vi "FTW-SEQ-Destroy.vi"(1 "FTW Job Sequencer":refnum<class "FTW-JobSequencer.lvclass">) -> ()   [LabVIEW 2012, in "FTW-Actor.lvlib" / "FTW-JobSequencer.lvclass"]
uses:
  FTW-JobSequencer.lvclass
panel:
  # "Inputs"
  # "Outputs"
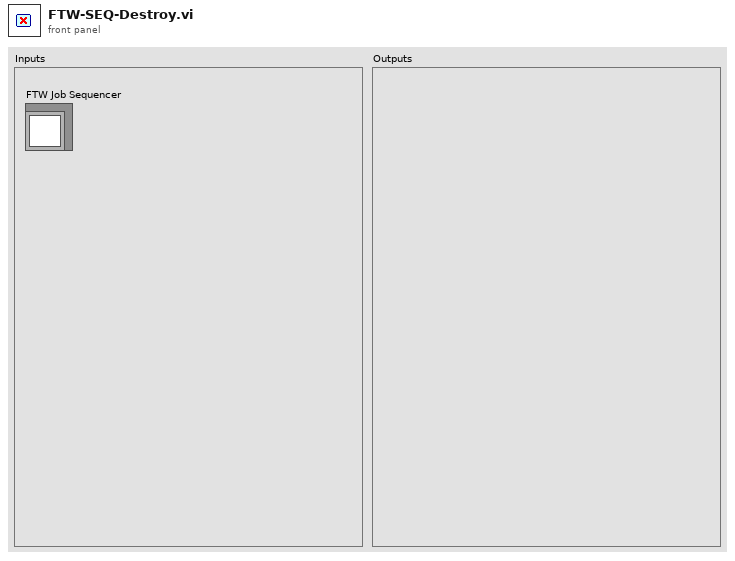
[diagram p1: front panel]
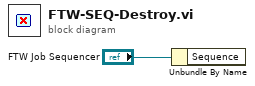
[diagram p0: block diagram]
diagram:
  n1 = Unbundle By Name("FTW Job Sequencer") -> ()  [unwired: 1 out]
